vi "Variant_ListElements.vi"(11 "Variant":variant) -> (1 "Has Elements":bool, 2 "element names":string[](array[string]), 3 "Variant dup":variant, 4 "Event Class":string[](array[string]))   [LabVIEW 2020, in "OpenVariant.lvlib"]
uses:
  OpenVariant.lvlib
  _built_ppls/OpenDescriptor.lvlibp
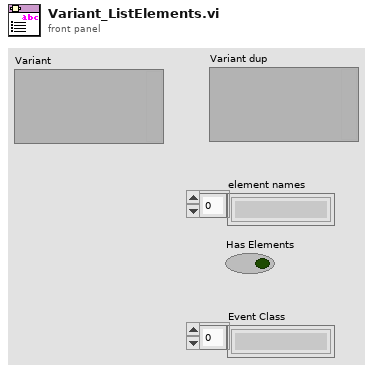
[diagram p1: front panel]
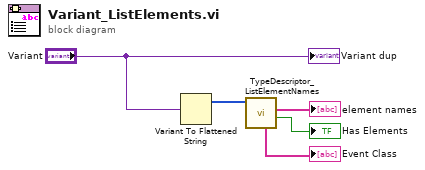
[diagram p0: block diagram]
diagram:
  n1 = Variant To Flattened String(Variant="Variant") -> (1:w4:i16[])  [unwired: 1 out]
  n2 = call "TypeDescriptor_ListElementNames.vi"("type descriptor"=w4) -> ("Has Elements"=→"Has Elements":bool, "element names"=→"element names":string[], "Event Class"=→"Event Class":string[])  [unwired: 7 in, 1 out]
  "Variant dup" <- "Variant"
